vi "Turn on Display.vi"(6 "chip select  (1st chip)":enum16{"1st chip", "2nd chip"}(ring), 8 "error in (no error)":errorcluster, 9 "cursor option":T1(ring)=enum."cursor on & no blink", 10 "display on?":bool=TRUE, 11 "HD44780 in":refnum<class "HD44780.lvclass">) -> (0 "error out":errorcluster, 3 "HD44780 out":refnum<class "HD44780.lvclass">)   [LabVIEW 2017, in "HD44780.lvclass"]
uses:
  HD44780.lvclass
  HD44780.lvclass/HD44780.ctl
  Common/HD44780 Common.lvlib
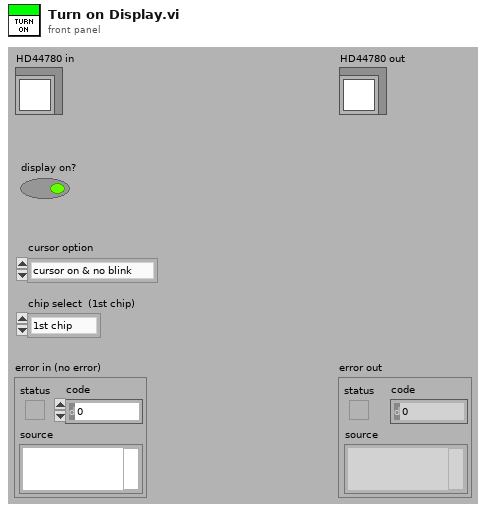
[diagram p1: front panel]
types:
  T1 = enum8{"cursor off", "cursor on & no blink", "cursor on & blink"}
  T2 = typedef "HD44780 Common.lvlib/cluster of class private data.ctl" = cluster{"FPGA VI Reference":refnum<k20>, "device index":i8, "screen size":T3, "font size":T4, "auto wrap":bool, "alignment":T5, "number of line":T6, "shift 0":i8, "entry mode 0":T7, "shift 1":i8, "entry mode 1":T7}
  T3 = typedef "HD44780 Common.lvlib/screen size.ctl" = enum8{"8x1", "8x2", "12x4", "16x1", "16x2", "16x4", "20x1", "20x2", "20x4", "24x1", "24x2", "40x2", "40x4"}
  T4 = typedef "HD44780 Common.lvlib/font size.ctl" = enum8{"5x8", "5x10"}
  T5 = typedef "HD44780 Common.lvlib/alignment.ctl" = enum16{"None", "Left", "Center", "Right"}
  T6 = typedef "HD44780 Common.lvlib/line number.ctl" = enum8{"1 line", "2 lines"}
  T7 = typedef "HD44780 Common.lvlib/entry mode.ctl" = enum8{"increment & no shift", "increment & shift", "decrement & no shift", "decrement & shift"}
  T8 = cluster{"FPGA VI Reference":refnum<k20>, "device index":i8, "screen size":enum8{"8x1", "8x2", "12x4", "16x1", "16x2", "16x4", "20x1", "20x2", "20x4", "24x1", "24x2", "40x2", "40x4"}, "font size":enum8{"5x8", "5x10"}, "auto wrap":bool, "alignment":enum16{"None", "Left", "Center", "Right"}, "number of line":enum8{"1 line", "2 lines"}, "shift 0":i8, "entry mode 0":enum8{"increment & no shift", "increment & shift", "decrement & no shift", "decrement & shift"}, "shift 1":i8, "entry mode 1":enum8{"increment & no shift", "increment & shift", "decrement & no shift", "decrement & shift"}}
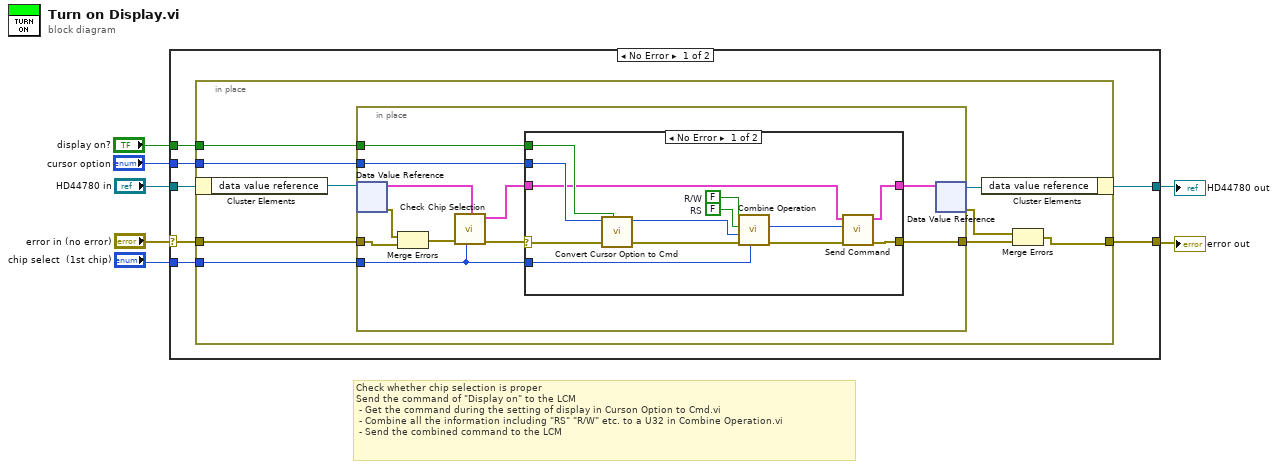
[diagram p0: block diagram]
diagram:
  # "Check whether chip selection is proper\nSend the command of \"Display on\" to the LCM \n - Get the command during the setting of display in Curson Option to Cmd.vi\n - Combine all the information including \"RS\" \"R/W\" etc. to a U32 in Combine Operation.vi \n - Send the combined command to the LCM"
  n1 = case shown="No Error" "error in (no error)" {
    selector: "error in (no error)" -> [w10 w49]
    tunnel: [w14 w49] -> w7
    tunnel: "chip select  (1st chip)" -> [w13 _]
    tunnel: "HD44780 in" -> [w12 w50]
    tunnel: [w11 w50] -> w4
    tunnel: "cursor option" -> [w9 _]
    tunnel: "display on?" -> [w8 _]
    frame No Error {
      n2 = in-place {
        in-place-border: [w18] -> w14
        in-place-border: w13 -> [w23]
        in-place-border: w10 -> [w17]
        in-place-border: w9 -> [w16]
        in-place-border: w8 -> [w15]
        n3 = in-place-cluster #1(w12) -> ("data value reference"=w22:refnum<data-value>)
        n4 = in-place {
          in-place-border: [w34] -> w19
          in-place-border: w23 -> [w29]
          in-place-border: w17 -> [w30]
          in-place-border: w16 -> [w27]
          in-place-border: w15 -> [w26]
          n5 = in-place-dvr #2(w22) -> (w33:T2, w31:errorcluster)
          n6 = Merge Errors(w31, w30) -> (w28:errorcluster)
          n7 = call "Check Chip Selection.vi"("chip select"=w29, "error in (no error)"=w28, "cluster of private data in"=w33) -> ("error out"=w24:errorcluster, "cluster of private data out"=w25:T8)  [unwired: 7 in]
          n8 = case shown="No Error" w24 {
            selector: w24 -> [w35 w47]
            tunnel: [w46 w47] -> w34
            tunnel: [w45 w48] -> w32
            tunnel: w29 -> [w44 _]
            tunnel: w27 -> [w43 _]
            tunnel: w26 -> [w42 _]
            tunnel: w25 -> [w36 w48]
            frame No Error {
              w37 = FALSE  # RS
              w41 = FALSE  # R/W
              n9 = call "Convert Cursor Option to Cmd.vi"("display option (on)"=w42, "cursor option"=w43) -> ("Display On Cmd"=w40:u8)  [unwired: 9 in]
              n10 = call "Combine Operation.vi"("chip select  (1st chip)"=w44, "error in (no error)"=w35, "cmd/data"=w40, "RS"=w37, "R/W"=w41) -> ("error out"=w39:errorcluster, "output"=w38:u32)  [unwired: 5 in]
              n11 = call "Send Command.vi"("error in (no error)"=w39, "operation"=w38, "cluster of private data in"=w36) -> ("error out"=w46:errorcluster, "cluster of private data out"=w45:T8)  [unwired: 6 in, 1 out]
            }
            frame Error {
            }
          }
          n12 = in-place-dvr #2(w32) -> (w21:refnum<data-value>, w20:errorcluster)
        }
        n13 = in-place-cluster #1("data value reference"=w21) -> (w11:refnum<class "HD44780.lvclass">)
        n14 = Merge Errors(w20, w19) -> (w18:errorcluster)
      }
    }
    frame Error {
    }
  }
  "error out" <- w7
  "HD44780 out" <- w4
